vi "Led Off.vi"(8 "error in (no error)":errorcluster, 11 "index":i32) -> (0 "error out":errorcluster, 3 "index_out":i32)   [LabVIEW 2013, in "FEMTO_LUCI-10.lvlib"]
doc: "This function switches the LUCI-LED off."
uses:
  FEMTO_LUCI-10.lvlib
  LUCI_10.dll
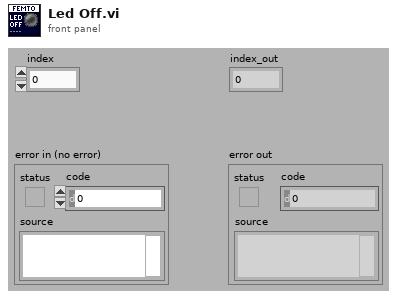
[diagram p1: front panel]
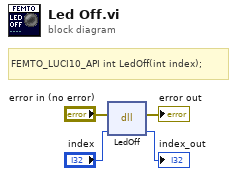
[diagram p0: block diagram]
diagram:
  # "FEMTO_LUCI10_API int LedOff(int index);"
  n1 = dll-call lib="C:/user/patrick/ppms_daq_femto/driver/LUCI_10.*" fn="LedOff"(error in="error in (no error)", "index"="index") -> (error out=→"error out":errorcluster, "index"=→"index_out":i32)  [unwired: 2 in, 2 out]
